vi "Begin.vi"(8 "error in (no error)":errorcluster, 10 "Settings":variant, 11 "Elevator in":refnum<class "Elevator.lvclass">) -> (0 "error out":errorcluster, 3 "Elevator out":refnum<class "Elevator.lvclass">)   [LabVIEW 2019, in "Elevator.lvlib" / "Elevator.lvclass"]
doc: "Use this VI to init the motors for the elevator"
uses:
  Elevator.lvclass
  Elevator.lvclass/Elevator.ctl
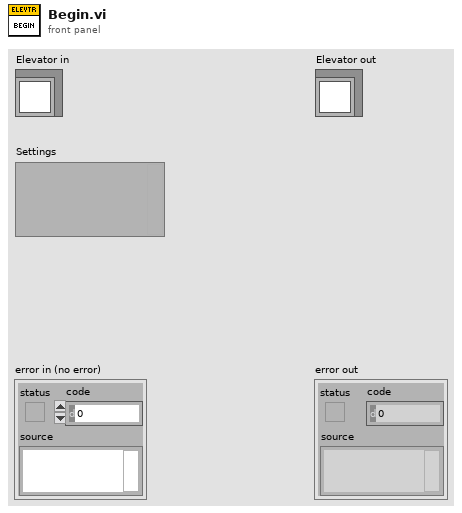
[diagram p1: front panel]
types:
  T1 = typedef "Elevator.lvlib/Elevator.lvclass/Elevator IDs.ctl" = cluster{"Wrist":u8, "Left Master":u8, "Left Slave":u8, "Right Master":u8, "Right Slave":u8, "Vacumm Pump 1":u8, "Vacumm Pump 2":u8, "Elevator Linear Master":u8, "Elevator Linear Slave":u8}
  T2 = typedef "Elevator.lvlib/Elevator.lvclass/Elevator Constants.ctl" = cluster{"Arm Motion Magic Max Velocity":u32, "Arm Motion Magic Max Acceleration":u32, "Wrist Motion Magic Max Velocity":u32, "Wrist Motion Magic Max Acceleration":u32, "Elevator Linear Motion Magic Max Velocity":u32, "Elevator Linear Motion Magic Max Acceleration":u32, "Arm Gear Ratio":dbl, "Wrist Gear Ratio":dbl, "Elevator Linear Gear Ratio":dbl, "Arm Encoder ABS Value":i32, "Wrist Encoder ABS Value":i32}
  T3 = typedef "CTRE_Phoenix_MotorControl_SlotStructure.ctl" = cluster{"P":dbl, "I":dbl, "D":dbl, "F":dbl, "integralZone":dbl, "allowableClosedLoopError":i32, "maxIntegralAccumulator":dbl, "closedLoopPeakOutput":dbl, "closedLoopPeriod":i32}
  T4 = typedef "Elevator.lvlib/Elevator.lvclass/Arm Position Values.ctl" = cluster{"C0 Arm":dbl, "C1 Arm":dbl, "C2 Arm":dbl, "H1 Arm":dbl, "H2 Arm":dbl, "C0 Wrist":dbl, "C1 Wrist ":dbl, "C2 Wrist":dbl, "H1 Wrist":dbl, "H2 Wrist":dbl, "Deploy Arm":dbl, "Deploy Wrist":dbl, "Climb Arm":dbl, "Climb Wrist":dbl, "Stowed Arm":dbl, "Stowed Wrist":dbl, "CS":dbl, "C0":dbl, "C1":dbl, "C2":dbl, "C3":dbl, "H0":dbl, "H1":dbl, "H2":dbl}
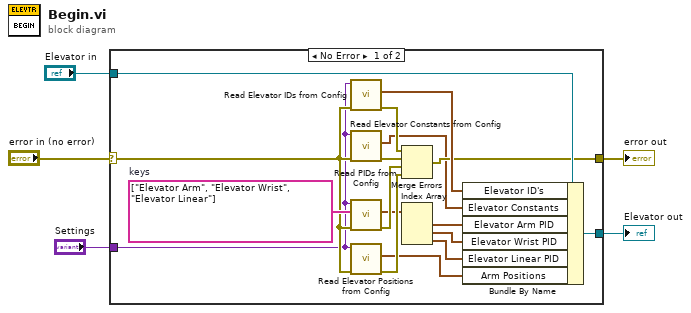
[diagram p0: block diagram]
diagram:
  n1 = case shown="No Error" "error in (no error)" {
    selector: "error in (no error)" -> [w9 w24]
    tunnel: [w18 w24] -> w4
    tunnel: [w21 w23] -> w2
    tunnel: "Elevator in" -> [w22 w23]
    tunnel: "Settings" -> [w8 _]
    frame No Error {
      w12 = string[] ["Elevator Arm", "Elevator Wrist", "Elevator Linear"]  # keys
      n2 = call "Read Elevator IDs from Config.vi"("error in (no error)"=w9, "Settings in"=w8) -> ("error out"=w19:errorcluster, "Elevator ID's"=w20:T1)  [unwired: 7 in, 1 out]
      n3 = call "Read Elevator Constants from Config.vi"("error in (no error)"=w9, "Settings"=w8) -> ("error out"=w10:errorcluster, "Elevator Constants"=w7:T2)  [unwired: 7 in, 1 out]
      n4 = call "Read PIDs from Config.vi"("error in (no error)"=w9, "keys"=w12, "Settings"=w8) -> ("error out"=w15:errorcluster, "Array"=w11:T3[])  [unwired: 6 in, 1 out]
      n5 = call "Read Elevator Positions from Config.vi"("error in (no error)"=w9, "Settings"=w8) -> ("error out"=w17:errorcluster, "Arm Positions"=w16:T4)  [unwired: 7 in, 1 out]
      n6 = Merge Errors(w19, w10, w15, w17) -> (w18:errorcluster)
      n7 = Index Array(array=w11) -> (element #1=w14:T3, element #2=w13:T3, element #3=w6:T3)  [unwired: 3 in]
      n8 = Bundle By Name(cluster=w22, "Elevator ID's"=w20, "Elevator Constants"=w7, "Elevator Arm PID"=w14, "Elevator Wrist PID"=w13, "Elevator Linear PID"=w6, "Arm Positions"=w16) -> (w21:refnum<class "Elevator.lvclass">)
    }
    frame Error {
    }
  }
  "error out" <- w4
  "Elevator out" <- w2
